vi "BGA244_mode_HeAir.vi"(8 "error in":errorcluster, 11 "VISA in":refnum<visa-resource-name>="COM24") -> (0 "error out":errorcluster, 1 "gas 2":string, 2 "gas 1":string, 3 "VISA out":refnum<visa-resource-name>, 4 "status":bool, 5 "mode":string)   [LabVIEW 2019]
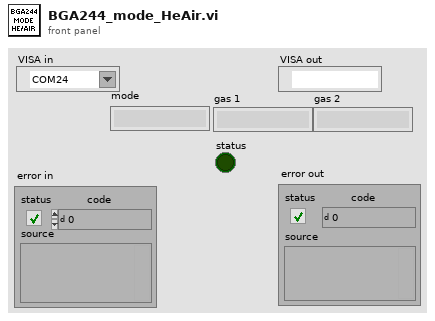
[diagram p1: front panel]
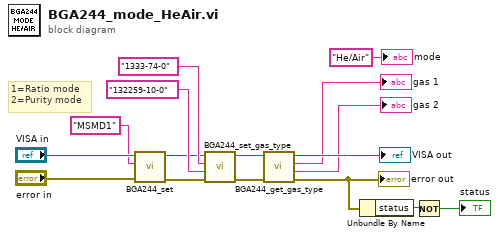
[diagram p0: block diagram]
diagram:
  # "1=Ratio mode\n2=Purity mode"
  n1 = call "BGA244_set.vi"("error in"="error in", "string in"="MSMD1", "VISA in"="VISA in") -> ("error out"=w9:errorcluster, "VISA out"=w2:refnum<visa-resource-name>)  [unwired: 7 in]
  n2 = call "BGA244_set_gas_type.vi"("error in"=w9, "gas 2"="132259-10-0", "gas 1"="1333-74-0", "VISA in"=w2) -> ("error out"=w8:errorcluster, "VISA out"=w7:refnum<visa-resource-name>)  [unwired: 5 in, 1 out]
  n3 = call "BGA244_get_gas_type.vi"("error in"=w8, "VISA in"=w7) -> ("error out"=w6:errorcluster, "gas 2"=→"gas 2":string, "gas 1"=→"gas 1":string, "VISA out"=→"VISA out":refnum<visa-resource-name>)  [unwired: 5 in, 1 out]
  "error out" <- w6
  n4 = Unbundle By Name(w6) -> ("status"=w14:bool)
  n5 = Not(x=w14) -> (.not. x?=→"status":bool)
  "mode" <- "He/Air" ("mode")
